vi "Error 5027.vi"(8 "error in (no error)":errorcluster, 10 "Method Name":string) -> (0 "error out":errorcluster)   [LabVIEW 2019, in "gRPC Template Creation Utility.lvlib"]
uses:
  gRPC Template Creation Utility.lvlib
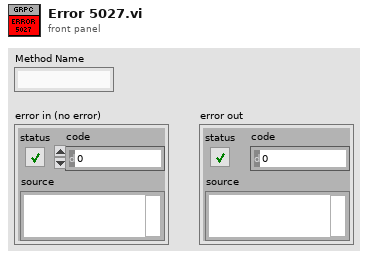
[diagram p1: front panel]
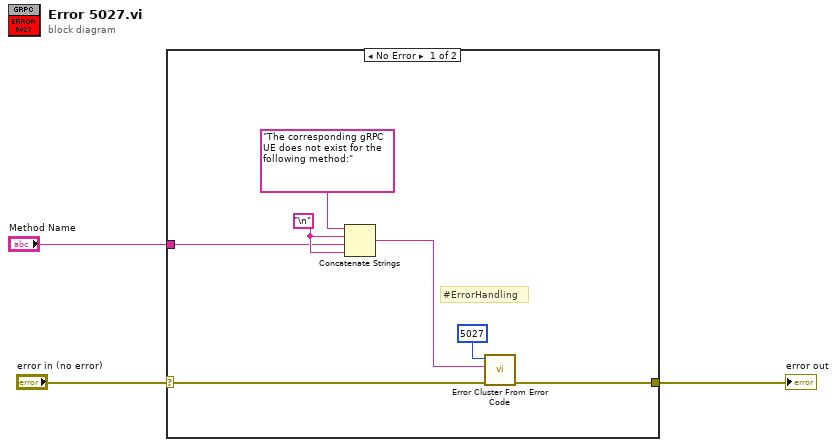
[diagram p0: block diagram]
diagram:
  n1 = case shown="No Error" "error in (no error)" {
    selector: "error in (no error)" -> [w4 w11]
    tunnel: "Method Name" -> [w9 _]
    tunnel: [w5 w11] -> w2
    frame No Error {
      w10 = "\n"
      # "#ErrorHandling"
      n2 = Concatenate Strings("The corresponding gRPC UE does not exist for the following method:" ("error message (\"\")"), w10, w9, w10) -> (w8:string)
      n3 = call <vilib>:"Error Cluster From Error Code.vi"("error in (no error)"=w4, "error message (\"\")"=w8, "error code (0)"=5027) -> ("error out"=w5:errorcluster)  [unwired: 6 in]
    }
    frame Error {
    }
  }
  "error out" <- w2
